vi "AFM_Driver_Manager.CreateEvents.vi"(8 "error in (no error)":errorcluster) -> (0 "error out":errorcluster, 3 "Events Cluster":T1)   [LabVIEW 2019, in "AFM_Driver_Manager.lvclass"]
uses:
  AFM_Driver_Manager.lvclass
  <userlib>/LevyLab/Relay Box/Typedefs/Resistor--enum.ctl
  <userlib>/LevyLab/Relay Box/Relay-Box.lvclass
  AFM_Driver_Manager.PublicMethods.ctl
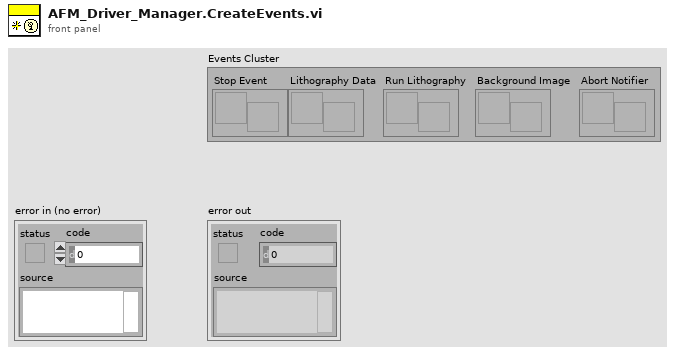
[diagram p1: front panel]
types:
  T1 = typedef "AFM_Driver_Manager.lvclass/AFM_Driver_Manager.PublicMethods.ctl" = cluster{"Stop Event":refnum<user-event>, "Lithography Data":refnum<user-event>, "Run Lithography":refnum<user-event>, "Background Image":refnum<user-event>, "Abort Notifier":refnum<user-event>}
  T2 = typedef "Relay-Box.lvclass/Resistor--enum.ctl" = enum16{"open", "discharge tip", "0 ohms", "100k ohm", "10M ohm", "1G ohm"}
  T3 = cluster{"Name":string, "Litho":cluster{"X":dbl, "Y":dbl, "Speed":dbl, "Voltage":dbl}[], "Set Resistance":T2, "Meta":variant}[]
  T4 = cluster{"VI Refnum":refnum<vi>, "Path":path, "Name":string, "Events":T1}[]
  T5 = cluster{"VI Refnum":refnum<vi>, "Path":path, "Name":string, "Events":T1}
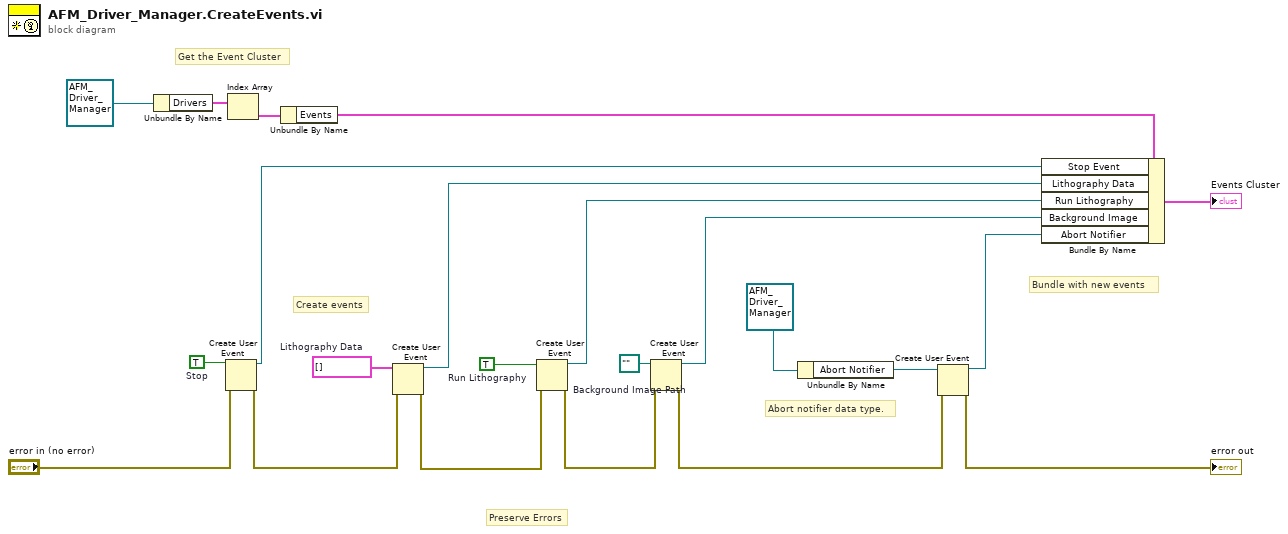
[diagram p0: block diagram]
diagram:
  w1 = T3 []  # Lithography Data
  w9 = path ""  # Background Image Path
  w16 = TRUE  # Run Lithography
  w19 = TRUE  # Stop
  # "Abort notifier data type."
  # "Preserve Errors"
  # "Create events"
  # "Bundle with new events"
  # "Get the Event Cluster"
  n1 = Unbundle By Name(refnum<class "AFM_Driver_Manager.lvclass"> refnum ("AFM_Driver_Manager in")) -> ("Drivers"=w14:T4)
  n2 = Create User Event(user event datatype=w19, error in="error in (no error)") -> (user event=w20:refnum<user-event>, error out=w11:errorcluster)
  n3 = Index Array(array=w14) -> (element=w21:T5)  [unwired: 1 in]
  n4 = Unbundle By Name(w21) -> ("Events"=w18:T1)
  n5 = Create User Event(user event datatype=w1, error in=w11) -> (user event=w17:refnum<user-event>, error out=w12:errorcluster)
  n6 = Create User Event(user event datatype=w16, error in=w12) -> (user event=w15:refnum<user-event>, error out=w8:errorcluster)
  n7 = Create User Event(user event datatype=w9, error in=w8) -> (user event=w10:refnum<user-event>, error out=w5:errorcluster)
  n8 = Unbundle By Name(refnum<class "AFM_Driver_Manager.lvclass"> refnum ("AFM_Driver_Manager in")) -> ("Abort Notifier"=w6:refnum<notifier>)
  n9 = Create User Event(user event datatype=w6, error in=w5) -> (user event=w3:refnum<user-event>, error out=→"error out":errorcluster)
  n10 = Bundle By Name(cluster=w18, "Stop Event"=w20, "Lithography Data"=w17, "Run Lithography"=w15, "Background Image"=w10, "Abort Notifier"=w3) -> (→"Events Cluster":T1)
